vi "QuadratureCtr_CountIndexStates.vi"(8 "First Run?":bool, 9 "Reset":bool, 11 "Valid Index State?":bool) -> (2 "Index State Count":u16, 3 "Save State?":bool)   [LabVIEW 2014, in "SYSID.lvlib"]
doc: "This VI counts the number of valid index states a quadrature counter has reached. It also determines when a save on index state occurs. It was designed to be called as a subVI in a loop on a LabVIEW FPGA VI block diagram in conjuction with a quadrature counter supporting Save On Index mode.\n\nThis VI is marked as reentrant so that it can be placed multiple times on the block diagram. Duplicate logic will be created in the FPGA for each instance of this VI the block diagram.\n\n<B>Inputs:</B>\n<B>Valid Index State?</B> - This represents whether the quadrature counter is in a valid index state. Logic in the calling VI computes whether the counter is in a valid index state based on A, B, and Z signals.\n\n<B>Reset</B> - This control resets the index state count to zero and sets the save state to TRUE.\n\n<B>First Run?</B> - This control ensures that the initial index state count is zero and the initial save state is TRUE. The caller of this VI should wire a TRUE into this input for its first call and a FALSE for subsequent calls.\n\n<B>Outputs:</B>\n<B>Index State Count</B> - This is the number of index states that have occurred since the counter was started or since it was last reset. The count increments each time a new valid index state is reached.\n\n<B>Save State?</B> - This indicates when a save should take place for the quadrature counter's Save On Index mode. Save State? is TRUE when the counter initializes, when the counter resets, and when a new valid index state is reached."
uses:
  SYSID.lvlib
  <vilib>/rvi/Emulation/niFpgaSctlEmulationGetInTimedLoop.vi
  <vilib>/rvi/Emulation/niFpgaProcessEmulError.vi
panel:
  out "Index State register":bool
  # "Inputs"
  # "Registers"
  # "Outputs"
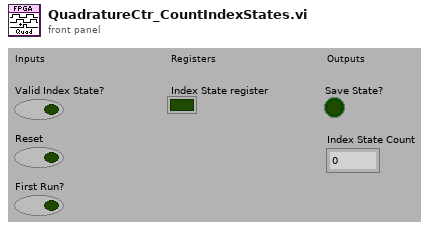
[diagram p1: front panel]
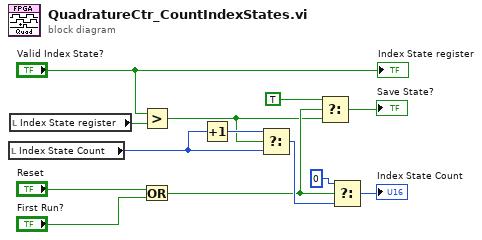
[diagram p0: block diagram]
diagram:
  n1 = local read "Index State Count"() -> (w7:u16)
  n2 = local read "Index State register"() -> (w9:bool)
  n3 = Greater?(x="Valid Index State?", y=w9) -> (0:w2:bool)
  n4 = Or(x="Reset", y="First Run?") -> (x .or. y?=w4:bool)
  n5 = Increment(x=w7) -> (x+1=w6:u16)
  n6 = Select(t=w6, s=w2, f=w7) -> (s? t:f=w10:u16)
  n7 = Select(t=TRUE, s=w4, f=w2) -> (s? t:f=→"Save State?":bool)
  n8 = Select(t=u16 0 ("I32"), s=w4, f=w10) -> (s? t:f=→"Index State Count":u16)
  "Index State register" <- "Valid Index State?"
